vi "DCMotor Example.vi"() -> ()   [LabVIEW 2012, in "Phidget DC Motor.lvlib"]
uses:
  <instrlib>/Phidgets/Phidget DC Motor/Phidget DC Motor.lvlib
  <instrlib>/Phidgets/Phidget DC Motor/Public/DCMotorStart.vi
  <instrlib>/Phidgets/Phidget DC Motor/Public/DCMotorClose.vi
  <instrlib>/Phidgets/Phidget Common/Phidget Common.lvlib
panel:
  in  "Acceleration":dbl=1.0
  in  "Velocity":dbl(slide) caption="Duty Cycle" scale=-1.0..1.0
  in  "stop":bool
  out "Current Velocity":dbl caption="Duty Cycle Return"
  in  "Device Info":T1={"Serial Number"=-1, "Channel"=0, "Port"=0}
  out "Attached?":bool
  out "Serial Number Return":i32
  out "error out":errorcluster
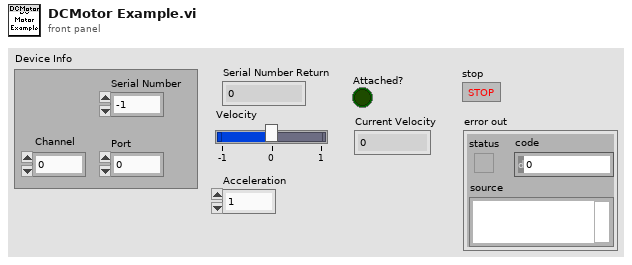
[diagram p1: front panel]
types:
  T1 = cluster{"Serial Number":i32, "Channel":i32, "Port":i32}
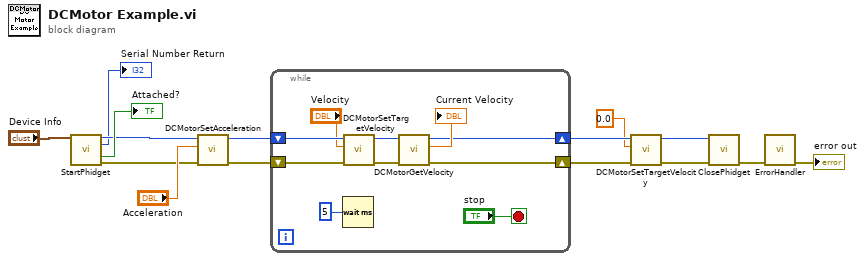
[diagram p0: block diagram]
diagram:
  n1 = call-poly <instrlib>:"StartPhidget.vi"("Device Info"="Device Info") -> ("Phidget ID"=w9:u64, "Serial Number Return"=→"Serial Number Return":i32, "Attached?"=→"Attached?":bool, "error out"=w2:errorcluster)  [unwired: 11 in]
  n2 = call <instrlib>:"DCMotorSetAcceleration.vi"("error in (no error)"=w2, "Acceleration"="Acceleration", "Device In"=w9) -> ("error out"=w11:errorcluster, "Device Out"=w12:u64)  [unwired: 6 in]
  n3 = while {
    shift-right: [w17] -> w8
    shift-left: w12 -> [w20]
    shift-right: [w16] -> w7
    shift-left: w11 -> [w19]
    stop <- "stop" stop-if-true
    n4 = Wait (ms)(milliseconds to wait=u32 5) -> ()  [unwired: 1 out]
    n5 = call <instrlib>:"DCMotorSetTargetVelocity.vi"("error in (no error)"=w19, "Velocity"="Velocity", "Device In"=w20) -> ("error out"=w22:errorcluster, "Device Out"=w21:u64)  [unwired: 6 in]
    n6 = call <instrlib>:"DCMotorGetVelocity.vi"("error in (no error)"=w22, "Device In"=w21) -> ("error out"=w16:errorcluster, "Velocity"=→"Current Velocity":dbl, "Device Out"=w17:u64)  [unwired: 6 in]
  }
  n7 = call <instrlib>:"DCMotorSetTargetVelocity.vi"("error in (no error)"=w7, "Velocity"=0.0 ("Velocity Limit"), "Device In"=w8) -> ("error out"=w6:errorcluster, "Device Out"=w5:u64)  [unwired: 6 in]
  n8 = call-poly <instrlib>:"ClosePhidget.vi"("error in"=w6, "Device In"=w5) -> ("error out"=w15:errorcluster)  [unwired: 9 in]
  n9 = call <instrlib>:"ErrorHandler.vi"("error in"=w15) -> ("error out"=→"error out":errorcluster)  [unwired: 9 in, 1 out]
